vi "DownloadRuntime.vi"(8 "error in":errorcluster, 11 "Downloader in":refnum<class "Downloader.lvclass">) -> (0 "error out":errorcluster, 3 "Downloader out":refnum<class "Downloader.lvclass">)   [LabVIEW 2014, in "Raspberry Pi Compatible Compiler for LabVIEW.lvlib" / "Downloader.lvclass"]
uses:
  Downloader.lvclass
  Downloader.lvclass/Downloader.ctl
  MessageBox/MessageBox.lvclass
  Websocket/Websocket.lvlib
  Download/RasPiDownloader.lvlib
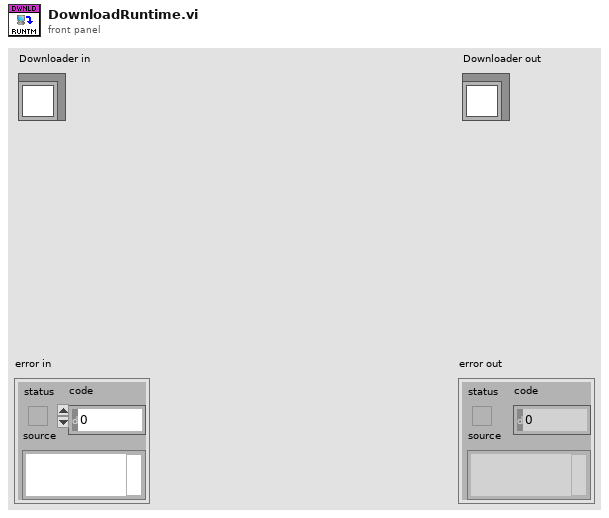
[diagram p1: front panel]
types:
  T1 = typedef "Raspberry Pi Compatible Compiler for LabVIEW.lvlib/RasPiDownloader.lvlib/RuntimeVersion.ctl" = cluster{"Major":i32, "Minor":i32, "Build":i32, "Revision":i32}
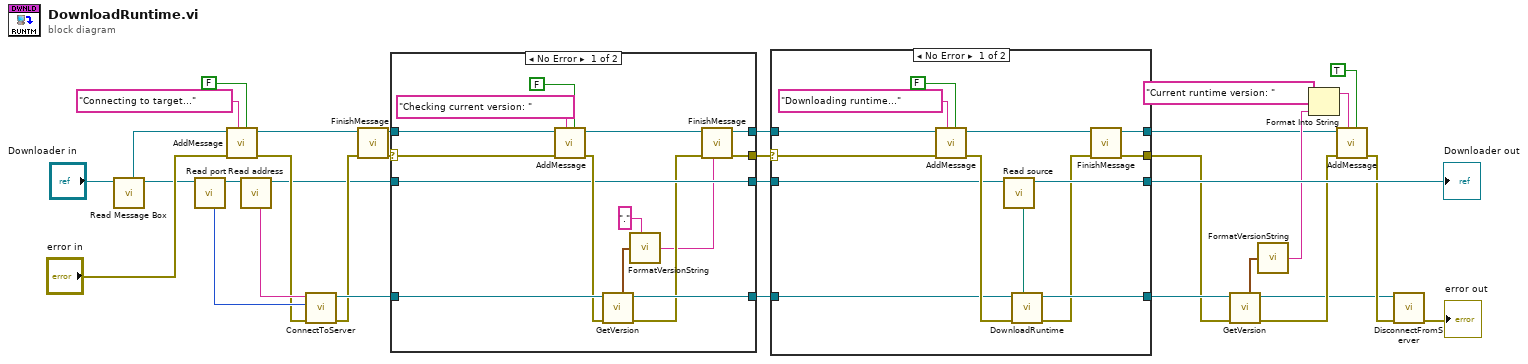
[diagram p0: block diagram]
diagram:
  n1 = call "Read Message Box.vi"("Downloader in"="Downloader in") -> ("Downloader out"=w26:refnum<class "Downloader.lvclass">, "Message Box"=w32:refnum<class "MessageBox.lvclass">)  [unwired: 7 in]
  n2 = call "Read port.vi"("Downloader in"=w26) -> ("Downloader out"=w24:refnum<class "Downloader.lvclass">, "port"=w28:u16)  [unwired: 7 in]
  n3 = call "AddMessage.vi"("add newline"=FALSE, "message"="Connecting to target...", "error in"="error in", "MessageBox in"=w32) -> ("error out"=w25:errorcluster, "MessageBox out"=w10:refnum<class "MessageBox.lvclass">)  [unwired: 4 in]
  n4 = call "Read address.vi"("Downloader in"=w24) -> ("Downloader out"=w5:refnum<class "Downloader.lvclass">, "address"=w27:string)  [unwired: 7 in]
  n5 = call "ConnectToServer.vi"("error in"=w25, "port"=w28, "address"=w27) -> ("error out"=w8:errorcluster, "connection ID"=w17:refnum<k5>)  [unwired: 5 in, 2 out]
  n6 = call "FinishMessage.vi"("error in"=w8, "MessageBox in"=w10) -> ("error out"=w9:errorcluster, "MessageBox out"=w7:refnum<class "MessageBox.lvclass">)  [unwired: 6 in]
  n7 = case shown="No Error" w9 {
    selector: w9 -> [w40 w51]
    tunnel: [w35 w52] -> w4
    tunnel: w17 -> [w46 w50]
    tunnel: [w36 w51] -> w3
    tunnel: [w43 w50] -> w16
    tunnel: w7 -> [w41 w52]
    tunnel: [w39 w49] -> w6
    tunnel: w5 -> [w39 w49]
    frame No Error {
      n8 = call "AddMessage.vi"("add newline"=FALSE, "message"="Checking current version: ", "error in"=w40, "MessageBox in"=w41) -> ("error out"=w45:errorcluster, "MessageBox out"=w38:refnum<class "MessageBox.lvclass">)  [unwired: 4 in]
      n9 = call "GetVersion.vi"("error in"=w45, "connection ID"=w46) -> ("error out"=w37:errorcluster, "connection ID out"=w43:refnum<k5>, "Version"=w44:T1)  [unwired: 5 in]
      n10 = call "FormatVersionString.vi"("Version"=w44, "delimiter"=".") -> ("Version string"=w34:string)  [unwired: 1 in]
      n11 = call "FinishMessage.vi"("no error"=w34, "error in"=w37, "MessageBox in"=w38) -> ("error out"=w36:errorcluster, "MessageBox out"=w35:refnum<class "MessageBox.lvclass">)  [unwired: 5 in]
    }
    frame Error {
    }
  }
  n12 = case shown="No Error" w3 {
    selector: w3 -> [w57 w69]
    tunnel: w4 -> [w65 w70]
    tunnel: [w55 w70] -> w2
    tunnel: [w54 w69] -> w1
    tunnel: [w62 w68] -> w20
    tunnel: w16 -> [w61 w67]
    tunnel: [w60 w67] -> w13
    tunnel: w6 -> [w58 w68]
    frame No Error {
      n13 = call "AddMessage.vi"("add newline"=FALSE, "message"="Downloading runtime...", "error in"=w57, "MessageBox in"=w65) -> ("error out"=w63:errorcluster, "MessageBox out"=w56:refnum<class "MessageBox.lvclass">)  [unwired: 4 in]
      n14 = call "Read source.vi"("Downloader in"=w58) -> ("Downloader out"=w62:refnum<class "Downloader.lvclass">, "source"=w59:path)  [unwired: 7 in]
      n15 = call "DownloadRuntime.vi"("Path"=w59, "error in"=w63, "WebSocket connection"=w61) -> ("error out"=w53:errorcluster, "WebSocket connection out"=w60:refnum<k5>)  [unwired: 5 in]
      n16 = call "FinishMessage.vi"("error in"=w53, "MessageBox in"=w56) -> ("error out"=w54:errorcluster, "MessageBox out"=w55:refnum<class "MessageBox.lvclass">)  [unwired: 6 in]
    }
    frame Error {
    }
  }
  "Downloader out" <- w20
  n17 = call "GetVersion.vi"("error in"=w1, "connection ID"=w13) -> ("error out"=w14:errorcluster, "connection ID out"=w12:refnum<k5>, "Version"=w15:T1)  [unwired: 5 in]
  n18 = call "FormatVersionString.vi"("Version"=w15) -> ("Version string"=w11:string)  [unwired: 2 in]
  n19 = Format Into String(initial string="Current runtime version: ", w11) -> (resulting string=w23:string)  [unwired: 2 in, 1 out]
  n20 = call "AddMessage.vi"("add newline"=TRUE, "message"=w23, "error in"=w14, "MessageBox in"=w2) -> ("error out"=w18:errorcluster)  [unwired: 4 in, 1 out]
  n21 = call "DisconnectFromServer.vi"("error in"=w18, "connection ID"=w12) -> ("error out"=→"error out":errorcluster)  [unwired: 7 in]
